vi "MoveShift.vi"(5 "max speed":dbl, 6 "Position":cluster{"X":dbl, "Y":dbl, "Theta":dbl}, 7 "Precision":dbl, 8 "theta":dbl, 9 "y shift":dbl, 10 "x shift":dbl, 11 "Error/Flow In":errorcluster) -> (0 "Position Out":cluster{"X":dbl, "Y":dbl, "Theta":dbl}, 3 "Error/Flow Out":errorcluster)   [LabVIEW 2018]
uses:
  <vilib>/Analysis/coordinate.llb/2D Cartesian Coordinate Rotation (Scalar).vi
  <vilib>/Analysis/coordinate.llb/2D Cartesian Coordinate Shift (Scalar).vi
  <vilib>/Analysis/NI_AALPro.lvlib
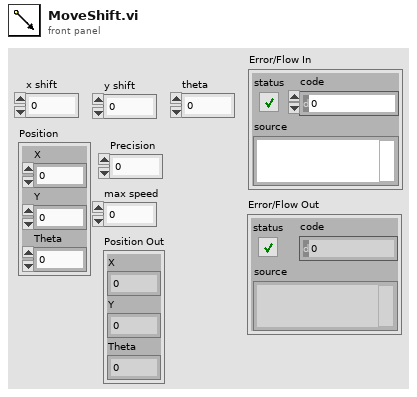
[diagram p1: front panel]
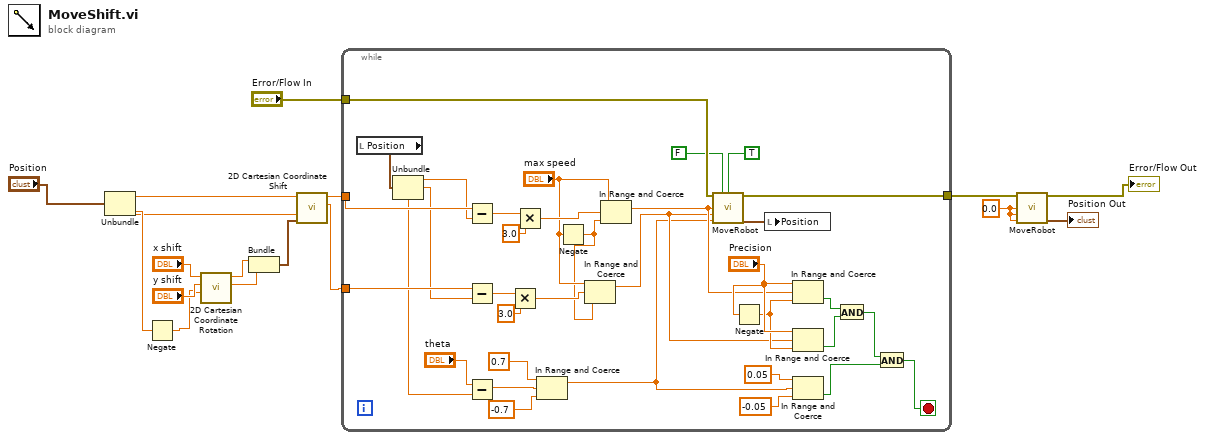
[diagram p0: block diagram]
diagram:
  w1 = 0.0 ("x (mm/s)")
  n1 = Unbundle("Position") -> ("X"=w10:dbl, "Y"=w9:dbl, "Theta"=w14:dbl)
  n2 = Negate(x=w14) -> (-x=w15:dbl)
  n3 = call-poly <vilib>:"2D Cartesian Coordinate Rotation.vi"("theta"=w15, "y"="y shift", "x"="x shift") -> ("y out"=w12:dbl, "x out"=w13:dbl)  [unwired: 6 in, 1 out]
  n4 = Bundle("x out"=w13, "y out"=w12) -> (w11:cluster{"x out":dbl, "y out":dbl})  [unwired: 1 in]
  n5 = call-poly <vilib>:"2D Cartesian Coordinate Shift.vi"("shift"=w11, "y"=w9, "x"=w10) -> ("y out"=w6:dbl, "x out"=w7:dbl)  [unwired: 6 in, 1 out]
  n6 = while {
    tunnel: w7 -> [w52]
    tunnel: w6 -> [w47]
    tunnel: "Error/Flow In" -> [w35]
    tunnel: [w32] -> w4
    stop <- w20 stop-if-true
    n7 = local read "Position"() -> (w19:cluster{"X":dbl, "Y":dbl, "Theta":dbl})
    n8 = Unbundle(w19) -> ("X"=w51:dbl, "Y"=w46:dbl, "Theta"=w39:dbl)
    n9 = Subtract(x=w52, y=w51) -> (x-y=w50:dbl)
    n10 = Subtract(x=w47, y=w46) -> (x-y=w44:dbl)
    n11 = Subtract(x="theta", y=w39) -> (x-y=w36:dbl)
    n12 = Multiply(x=w44, y=3.0) -> (x*y=w43:dbl)
    n13 = Multiply(x=w50, y=3.0) -> (x*y=w48:dbl)
    n14 = In Range and Coerce(upper limit=0.7, x=w36, lower limit=-0.7 ("upper limit")) -> (coerced(x)=w27:dbl)  [unwired: 1 out]
    n15 = Negate(x="max speed") -> (-x=w41:dbl)
    n16 = In Range and Coerce(upper limit="max speed", x=w43, lower limit=w41) -> (coerced(x)=w28:dbl)  [unwired: 1 out]
    n17 = In Range and Coerce(upper limit="max speed", x=w48, lower limit=w41) -> (coerced(x)=w29:dbl)  [unwired: 1 out]
    n18 = call "MoveRobot.vi"("Error/Flow In"=w35, "Reset"=FALSE, "Relative to Global Frame"=TRUE, "x (mm/s)"=w29, "y (mm/s)"=w28, "theta (rad/s)"=w27) -> ("Error/Flow Out"=w32:errorcluster, "Position"=w18:cluster{"X":dbl, "Y":dbl, "Theta":dbl})  [unwired: 8 in]
    n19 = Negate(x="Precision") -> (-x=w30:dbl)
    n20 = local write "Position"(w18) -> ()
    n21 = In Range and Coerce(upper limit="Precision", x=w29, lower limit=w30) -> (In Range?=w24:bool)  [unwired: 1 out]
    n22 = In Range and Coerce(upper limit="Precision", x=w28, lower limit=w30) -> (In Range?=w23:bool)  [unwired: 1 out]
    n23 = In Range and Coerce(upper limit=0.05, x=w27, lower limit=-0.05 ("upper limit")) -> (In Range?=w22:bool)  [unwired: 1 out]
    n24 = And(x=w24, y=w23) -> (x .and. y?=w21:bool)
    n25 = And(x=w21, y=w22) -> (x .and. y?=w20:bool)
  }
  n26 = call "MoveRobot.vi"("Error/Flow In"=w4, "x (mm/s)"=w1, "y (mm/s)"=w1, "theta (rad/s)"=w1) -> ("Error/Flow Out"=→"Error/Flow Out":errorcluster, "Position"=→"Position Out":cluster{"X":dbl, "Y":dbl, "Theta":dbl})  [unwired: 10 in]
